vi "Observe Data.vi"(6 "Time Stamp":timestamp, 8 "error in (no error)":errorcluster, 9 "Value":variant, 10 "Datum Name":string, 11 "BasicTerminalBinding in":refnum<class "BasicTerminalBinding.lvclass">) -> (0 "error out":errorcluster, 3 "BasicTerminalBinding out":refnum<class "BasicTerminalBinding.lvclass">)   [LabVIEW 2020, in "TestViewables.lvlib" / "BasicTerminalBinding.lvclass"]
doc: "观察数据"
uses:
  BasicTerminalBinding.lvclass
  modules/mva-viewable/Source/IViewable/IViewable/IViewable.lvclass
  BasicTerminalBinding.lvclass/BasicTerminalBinding.ctl
panel:
  out "x-y":dbl
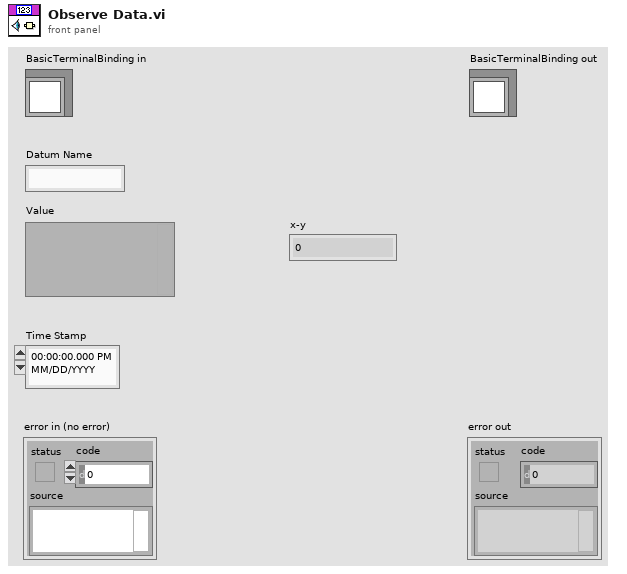
[diagram p1: front panel]
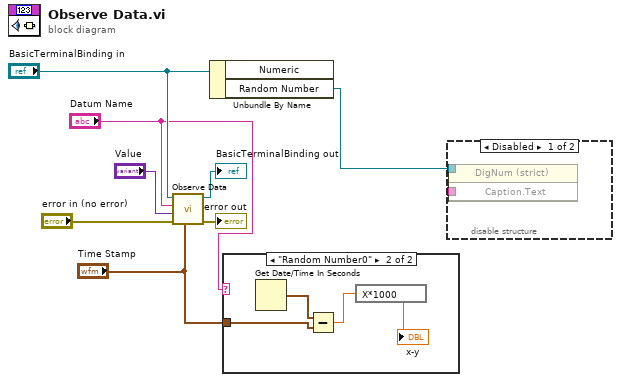
[diagram p0: block diagram]
diagram:
  n1 = call-parent "Observe Data.vi"("Time Stamp"="Time Stamp", "error in (no error)"="error in (no error)", "Value"="Value", "Datum Name"="Datum Name", "IObserver in"="BasicTerminalBinding in") -> ("error out"=→"error out":errorcluster, "IObserver out"=→"BasicTerminalBinding out":refnum<class "BasicTerminalBinding.lvclass">)  [unwired: 5 in]
  n2 = Unbundle By Name("BasicTerminalBinding in") -> ("Random Number"=w3:refnum<vi>)  [unwired: 1 out]
  n3 = case shown="\"Random Number0\"" "Datum Name" {
    tunnel: "Time Stamp" -> [_ w11]
    frame "False", Default {
    }
    frame "Random Number0" {
      n4 = Get Date/Time In Seconds() -> (seconds since 1Jan1904=w12:timestamp)
      n5 = Subtract(x=w12, y=w11) -> (x-y=w10:dbl)
      n6 = expression code="X*1000"(w10) -> (→"x-y":dbl)
    }
  }
  n7 = disable-structure shown="Disabled" {
    disable-tunnel: w3 -> [w14 _]
    disable-tunnel: _ -> [w13 _]
    frame Disabled {
      n8 = property class="DigNum (strict)"(reference=w14, "Caption.Text"=w13) -> ()  [unwired: 1 in, 2 out]
    }
    frame Enabled {
    }
  }
